vi "SENS_CORR_CSET_SEL_S.vi"(0 "VISA IN":refnum<visa-resource-name>, 1 "DEF or USER01...USER10":string, 5 "error in":errorcluster, 7 "Channel":i32) -> (14 "VISA Out":refnum<visa-resource-name>, 19 "error out":errorcluster)   [LabVIEW 2018, in "PNA-X.lvlib"]
doc: "SENSe<cnum>:CORRection:CSET[:SELect] <char> Superseded \n1695\n\nThis command is replaced by MMEM:LOAD \n(Read-Write) Restores a state file from memory. The file name is \"CSETx.cst\" where x is the user \nnumber assigned to <char>, and .cst specifies a cal set and instrument state. This is not the same \nsyntax as a file saved through the default choices from the front panel, which is \"at00x.cst\". For more \ninformation on the file naming syntax, see the MMEMory subsystem. Learn more about \nInstrument/Cal States. \nNote: This command does NOT select a Cal Set for a channel. To select a Cal Set, use \nSENS:CORR:CSET:ACTivate \nParameters \n<cnum> Any existing channel number. If unspecified, value is set to 1 \n<char> Choose from: \nDEF - Presets the analyzer \nUSER01 - Restores User01 calibration data \nUSER02 - Restores User02 calibration data \nthrough... \nUSER10 - Restores User10 calibration data \nExamples SENS:CORR:CSET DEF \nsense2:correction:cset:select user02 \nQuery Syntax SENSe<cnum>:CORRection:CSET[:SELect]? \nReturn Type Character \nDefault DEF"
uses:
  PNA-X.lvlib
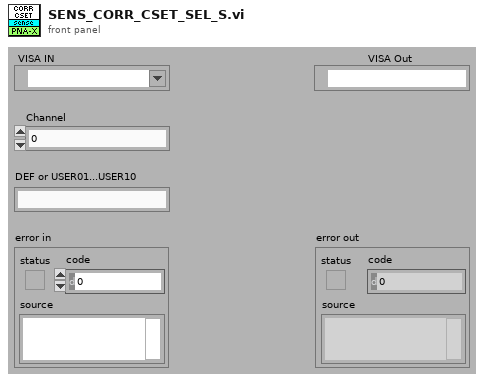
[diagram p1: front panel]
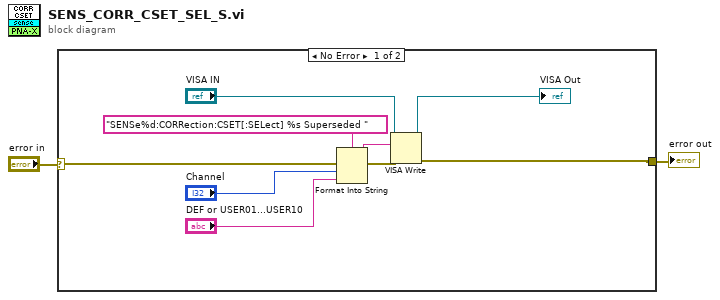
[diagram p0: block diagram]
diagram:
  n1 = case shown="No Error" "error in" {
    selector: "error in" -> [w11 w12]
    tunnel: [w6 w12] -> w1
    frame No Error {
      n2 = Format Into String(format string="SENSe%d:CORRection:CSET[:SELect] %s Superseded " ("Cmdline"), error in=w11, "Channel", "DEF or USER01...USER10") -> (resulting string=w9:string, error out=w10:errorcluster)  [unwired: 1 in]
      n3 = VISA Write(VISA resource name="VISA IN", write buffer=w9, error in (no error)=w10) -> (VISA resource name out=→"VISA Out":refnum<visa-resource-name>, error out=w6:errorcluster)  [unwired: 1 out]
    }
    frame Error {
    }
  }
  "error out" <- w1
